vi "_MISC_ Cursor2Mouse.vi"(8 "Error In":errorcluster, 9 "Cursor Index":i32, 10 "Coords":T1, 11 "WaveformGraph Ref":refnum<vi>) -> (0 "Error out":errorcluster, 3 "XY":cluster{"X":dbl, "Y":dbl})   [LabVIEW 2014]
uses:
  <vilib>/Utility/miscctls.llb/LVPoint32TypeDef.ctl
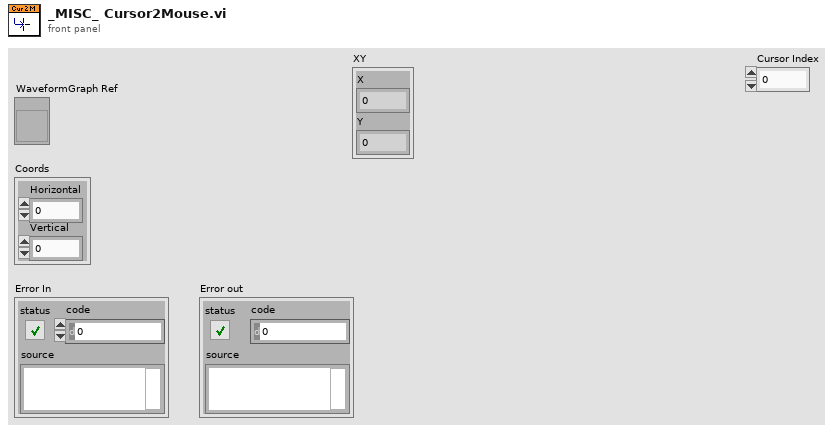
[diagram p1: front panel]
types:
  T1 = typedef "LVPoint32TypeDef.ctl" = cluster{"Horizontal":i32, "Vertical":i32}
  T2 = typedef "LVCursorListTypeDef.ctl" = cluster{"Name":string, "Color":u32, "Style":u8, "Point Style":u8, "Name Visible":bool, "Allow Drag":bool, "Cursor Mode":u32, "Plot":i32, "Index":i32, "Position":cluster{"X":dbl, "Y":dbl}, "X Scale":u32, "Y Scale":u32, "Watch Plots":i32[], "Watch All Plots":bool, "Plot Area":i32, "Label Offset":cluster{"X":dbl, "Y":dbl}}[]
  T3 = cluster{"Name":string, "Color":u32, "Style":u8, "Point Style":u8, "Name Visible":bool, "Allow Drag":bool, "Cursor Mode":u32, "Plot":i32, "Index":i32, "Position":cluster{"X":dbl, "Y":dbl}, "X Scale":u32, "Y Scale":u32, "Watch Plots":i32[], "Watch All Plots":bool, "Plot Area":i32, "Label Offset":cluster{"X":dbl, "Y":dbl}}
  T4 = cluster{"Name":string, "Color":u32, "Style":u8, "Point Style":u8, "Name Visible":bool, "Allow Drag":bool, "Cursor Mode":u32, "Plot":i32, "Index":i32, "Position":cluster{"X":dbl, "Y":dbl}, "X Scale":u32, "Y Scale":u32, "Watch Plots":i32[], "Watch All Plots":bool, "Plot Area":i32, "Label Offset":cluster{"X":dbl, "Y":dbl}}[]
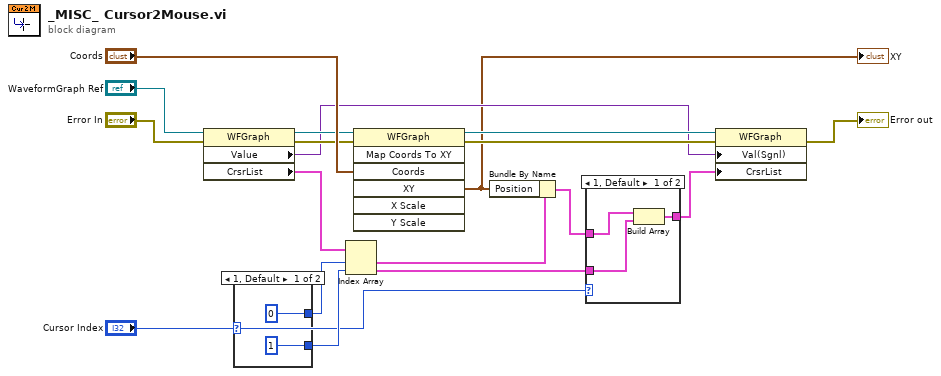
[diagram p0: block diagram]
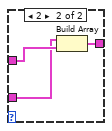
[diagram p2: hidden frame]
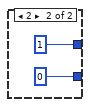
[diagram p3: hidden frame]
diagram:
  n1 = property class="WFGraph"(reference="WaveformGraph Ref", error in="Error In") -> (reference out=w5:refnum<vi>, error out=w6:errorcluster, "Value"=w2:variant, "CrsrList"=w15:T2)
  n2 = case shown="1, Default" "Cursor Index" {
    tunnel: [1 ("index") 0 ("index")] -> w14
    tunnel: [0 ("index") 1 ("index")] -> w13
    frame 1, Default {
    }
    frame 2 {
    }
  }
  n3 = Index Array(array=w15, index #1=w13, index #2=w14) -> (element #1=w12:T3, element #2=w9:T3)
  n4 = invoke class="WFGraph" method="Map Coords To XY"(reference=w5, error in=w6, "Coords"="Coords") -> (reference out=w4:refnum<vi>, error out=w3:errorcluster, "XY"=w1:cluster{"X":dbl, "Y":dbl})  [unwired: 4 in, 4 out]
  "XY" <- w1
  n5 = Bundle By Name(cluster=w12, "Position"=w1) -> (w10:T3)
  n6 = case shown="1, Default" "Cursor Index" {
    tunnel: w10 -> [w25 w28]
    tunnel: w9 -> [w24 w27]
    tunnel: [w23 w26] -> w8
    frame 1, Default {
      n7 = Build Array(w25, w24) -> (w23:T4)
    }
    frame 2 {
      n8 = Build Array(w27, w28) -> (w26:T4)
    }
  }
  n9 = property class="WFGraph"(reference=w4, error in=w3, "Val(Sgnl)"=w2, "CrsrList"=w8) -> (error out=→"Error out":errorcluster)  [unwired: 1 out]
